vi "Save Chunk.vi"(4 "Volatge Y":dbl[](array[numeric]), 6 "End of file":bool, 8 "error in (no error)":errorcluster, 9 "Voltage X":dbl[](array[numeric]), 10 "Frequency":dbl[](array[numeric]), 11 "Spectrum Recorder in":refnum<class "Spectrum Recorder too.lvclass">) -> (0 "error out":errorcluster, 1 "Valid path":bool, 2 "Acquired Result.lvclass":refnum<class "Acquired Result.lvclass">, 3 "Spectrum Recorder out":refnum<class "Spectrum Recorder too.lvclass">)   [LabVIEW 2016, in "Spectrum Recorder too.lvclass"]
uses:
  Spectrum Recorder too.lvclass
  C:/github/LabActor/Worker/Worker.lvclass
  C:/github/LabActor/Template Module/Template Module.lvclass
  C:/Program Files (x86)/National Instruments/LabVIEW 2016/vi.lib/ActorFramework/Actor/Actor.lvclass
  Results/Acquired Result/Acquired Result.lvclass
  Spectrum Recorder too.lvclass/Spectrum Recorder too.ctl
  Results/File Path Result/File Path Result.lvclass
  C:/github/LabActor/Results/Acquired Result/Acquired Result.lvclass
  Worker/Worker.lvclass/Worker.ctl
  <vilib>/ActorFramework/Actor/Actor.lvclass/Actor.ctl
  Controllers/Process Controller Messages/Update Plots Msg/Update Plots Msg.lvclass/Update Plots Msg.ctl
  <vilib>/ActorFramework/Message Enqueuer/Message Enqueuer.lvclass/Message Enqueuer.ctl
  Worker/Read Cycle count.vi
  Worker/Write Cycle count.vi
  Template Module/Read Reply to.vi
  <vilib>/ActorFramework/Message Enqueuer/Enqueue.vi
  Controllers/Process Controller Messages/Update Plots Msg/Update Plots Msg.lvclass
  C:/Program Files (x86)/National Instruments/LabVIEW 2016/vi.lib/ActorFramework/Message/Message.lvclass
  <vilib>/ActorFramework/Message Priority Queue/Priority Enqueue.vi
  Template Module Messages/Result Reply Msg/Result Reply Msg.lvclass
  <vilib>/ActorFramework/Actor/Actor.lvclass
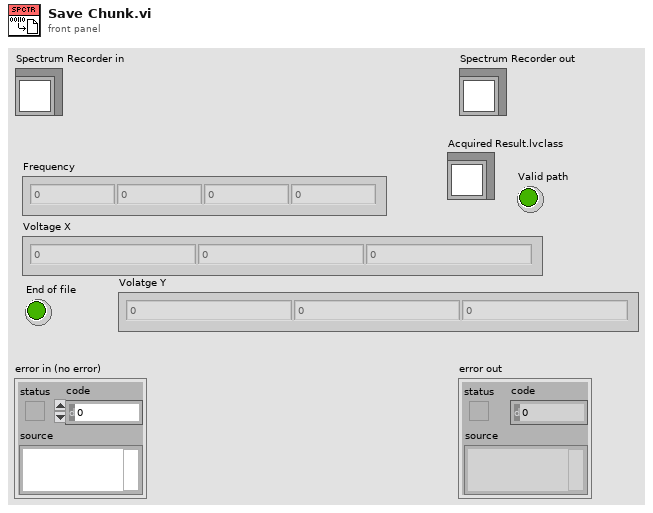
[diagram p1: front panel]
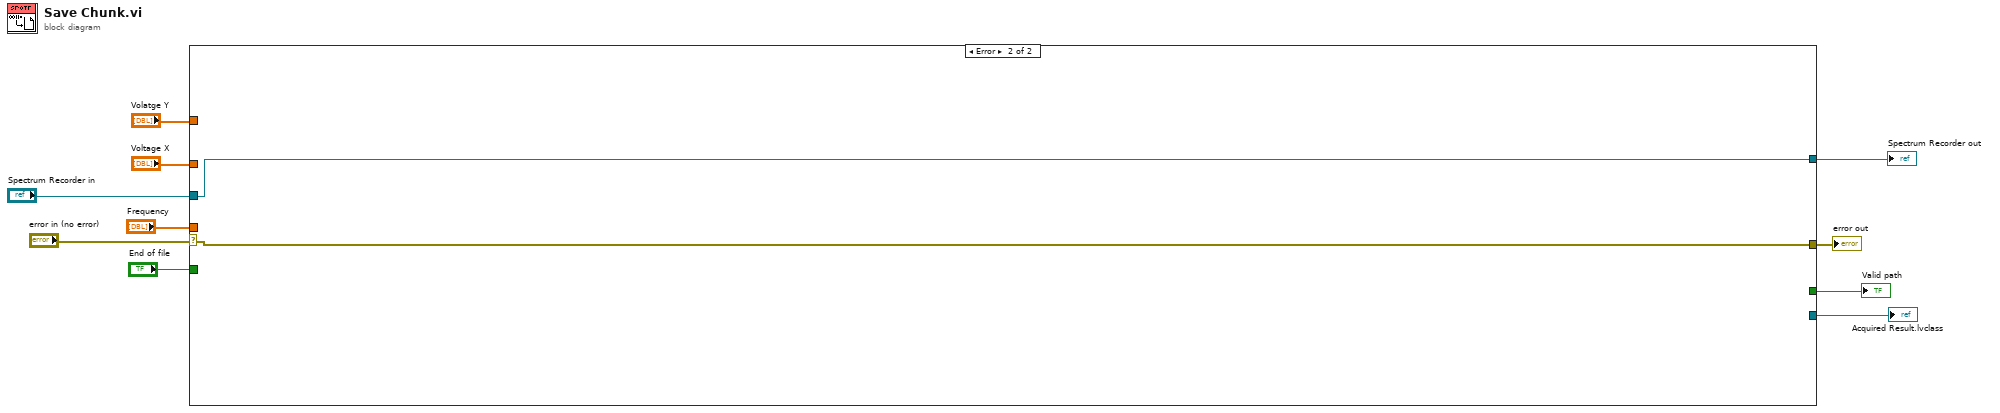
[diagram p0: block diagram]
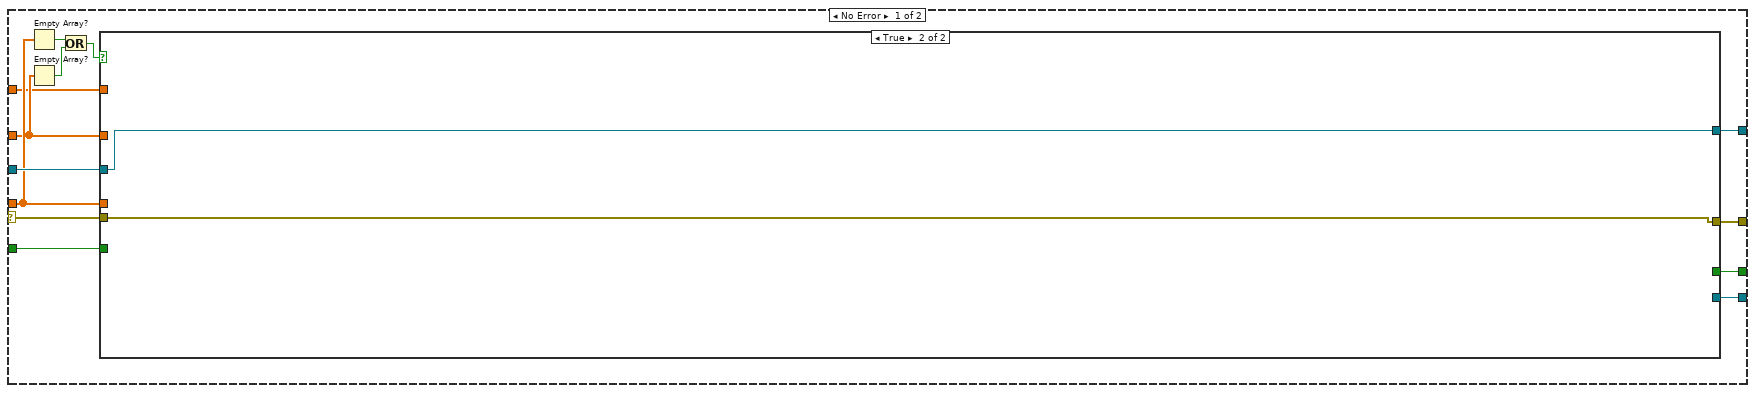
[diagram p2: hidden frame]
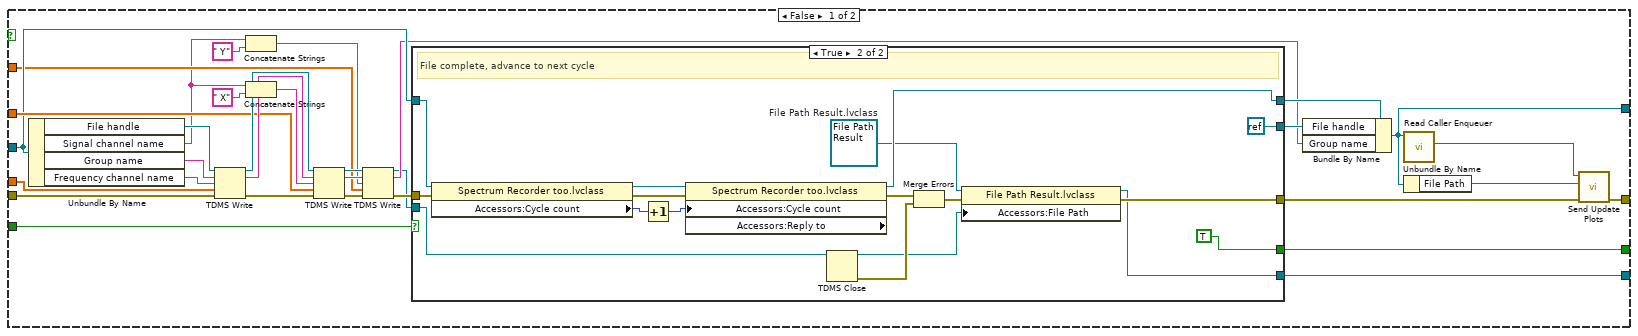
[diagram p3: hidden frame]
diagram:
  n1 = case shown="Error" "error in (no error)" {
    selector: "error in (no error)" -> [w21 w79]
    tunnel: [w20 w79] -> w9
    tunnel: [w22 w78] -> w7
    tunnel: "Spectrum Recorder in" -> [w23 w78]
    tunnel: "Voltage X" -> [w15 _]
    tunnel: "Frequency" -> [w16 _]
    tunnel: "End of file" -> [w14 _]
    tunnel: "Volatge Y" -> [w13 _]
    tunnel: [w12 _] -> w2
    tunnel: [w11 _] -> w1
    frame No Error {
      n2 = Empty Array?(array=w16) -> (empty?=w19:bool)
      n3 = Empty Array?(array=w15) -> (empty?=w18:bool)
      n4 = Or(x=w19, y=w18) -> (x .or. y?=w17:bool)
      n5 = case shown="True" w17 {
        tunnel: w15 -> [w48 _]
        tunnel: w16 -> [w52 _]
        tunnel: w23 -> [w45 w77]
        tunnel: [w27 w77] -> w22
        tunnel: w21 -> [w53 w76]
        tunnel: [w29 w76] -> w20
        tunnel: w14 -> [w46 _]
        tunnel: w13 -> [w37 _]
        tunnel: [w25 _] -> w12
        tunnel: [w24 _] -> w11
        frame False {
          n6 = Unbundle By Name(w45) -> ("File handle"=w55:refnum<k34>, "Signal channel name"=w32:string, "Group name"=w54:string, "Frequency channel name"=w47:string)
          n7 = TDMS Write(0:w55, 5:w54, 7:w47, 9:w52, 11:w53) -> (4:w50:refnum<k34>, 6:w49:string, 15:w51:errorcluster)  [unwired: 1 in, 1 out]
          n8 = Concatenate Strings(w32, " Y" ("string")) -> (w33:string)
          n9 = Concatenate Strings(w32, " X" ("string")) -> (w35:string)
          n10 = TDMS Write(0:w50, 5:w49, 7:w35, 9:w48, 11:w51) -> (4:w41:refnum<k34>, 6:w39:string, 15:w42:errorcluster)  [unwired: 1 in, 1 out]
          n11 = TDMS Write(0:w41, 5:w39, 7:w33, 9:w37, 11:w42) -> (4:w31:refnum<k34>, 6:w38:string, 15:w40:errorcluster)  [unwired: 1 in, 1 out]
          n12 = case shown="True" w46 {
            tunnel: w31 -> [w57 w75]
            tunnel: w40 -> [w56 w70]
            tunnel: [w56 w61] -> w28
            tunnel: w45 -> [w58 w71]
            tunnel: [w58 w68] -> w44
            tunnel: [w57 refnum<k0> refnum] -> w43
            tunnel: [_ w60] -> w25
            tunnel: [_ TRUE] -> w24
            frame False {
            }
            frame True {
              w64 = refnum<class "File Path Result.lvclass"> refnum  # File Path Result.lvclass
              # "File complete, advance to next cycle"
              n13 = property class="Spectrum Recorder too.lvclass"(reference=w71, error in=w70) -> (reference out=w74:refnum<class "Spectrum Recorder too.lvclass">, error out=w73:errorcluster, "Accessors:Cycle count"=w72:i32)
              n14 = Increment(x=w72) -> (x+1=w67:i32)
              n15 = property class="Spectrum Recorder too.lvclass" props=["Accessors:Cycle count", "Accessors:Reply to"](reference=w74, error in=w73, "Accessors:Cycle count"=w67) -> (reference out=w68:refnum<class "Spectrum Recorder too.lvclass">, error out=w69:errorcluster)  [unwired: 1 out]
              n16 = TDMS Close(11:w75) -> (0:w65:errorcluster, 3:w63:path)  [unwired: 1 in]
              n17 = Merge Errors(w69, w65) -> (w62:errorcluster)
              n18 = property class="File Path Result.lvclass"(reference=w64, error in=w62, "Accessors:File Path"=w63) -> (reference out=w60:refnum<class "File Path Result.lvclass">, error out=w61:errorcluster)
            }
          }
          n19 = Bundle By Name(cluster=w44, "File handle"=w43, "Group name"=w38) -> (w27:refnum<class "Spectrum Recorder too.lvclass">)
          n20 = call <vilib>:"Read Caller Enqueuer.vi"("Actor"=w27) -> ("Caller Enqueuer"=w30:refnum<class "Message Enqueuer.lvclass">)  [unwired: 10 in]
          n21 = Unbundle By Name(w27) -> ("File Path"=w26:path)
          n22 = call "Send Update Plots.vi"("error in (no error)"=w28, "File Path"=w26, "Message Enqueuer"=w30) -> ("error out"=w29:errorcluster)  [unwired: 7 in, 1 out]
        }
        frame True {
        }
      }
    }
    frame Error {
    }
  }
  "error out" <- w9
  "Spectrum Recorder out" <- w7
  "Acquired Result.lvclass" <- w2
  "Valid path" <- w1
